vi "EventSimulator.vi"() -> ()   [LabVIEW 2019, in "Mark 10 TSTM-DC.lvlib" / "Mark 10 Event Monitor.lvlib"]
uses:
  Mark 10 Event Monitor.lvlib
panel:
  in  "Type":enum16{"Tx", "Rx"}(ring)=enum."Rx"
  in  "Boolean":bool
  in  "String":string
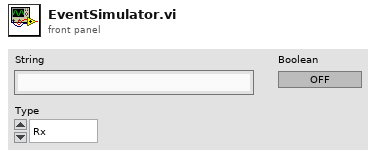
[diagram p1: front panel]
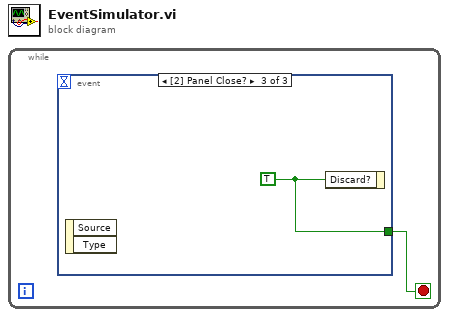
[diagram p0: block diagram]
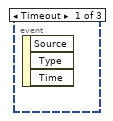
[diagram p2: hidden frame]
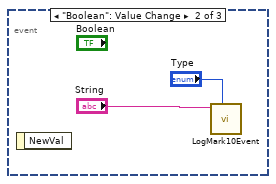
[diagram p3: hidden frame]
diagram:
  n1 = while {
    stop <- w1 stop-if-true
    n2 = event shown="[2] Panel Close?" {
      selector: _ -> [_ _ _]
      dyn-events: _ -> [_ _ _]
      timeout: _ -> [_ _ _]
      tunnel: [_ _ w4] -> w1
      event Timeout {
        n3 = event-data() -> ()  [unwired: 1 in, 3 out]
      }
      event "Boolean": Value Change {
        n4 = event-data() -> ()  [unwired: 1 in, 1 out]
        n5 = call "LogMark10Event.vi"("Type"="Type", "Event"="String") -> ()  [unwired: 9 in, 1 out]
      }
      event Panel Close? {
        w4 = TRUE ("Discard?")
        n6 = event-data() -> ()  [unwired: 1 in, 2 out]
        n7 = event-data("Discard?"=w4) -> ()  [unwired: 1 in, 1 out]
      }
    }
  }
